vi "例7-4(2).vi"() -> ()   [LabVIEW 2019]
panel:
  in  "端口":dbl=65511.0
  out "波形图（客户机）":dbl[](graph)
  in  "停止按钮":bool
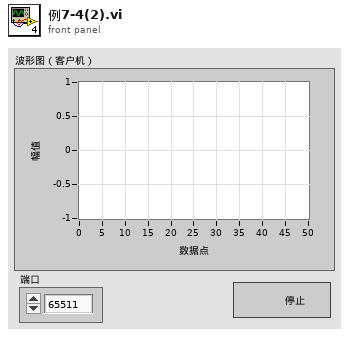
[diagram p1: front panel]
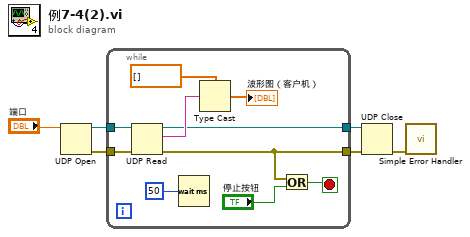
[diagram p0: block diagram]
diagram:
  n1 = UDP Open(11:"端口") -> (port=w6:refnum<k16>, 0:w5:errorcluster)  [unwired: 4 in, 1 out]
  n2 = while {
    tunnel: w6 -> [w16]
    tunnel: w5 -> [w15]
    tunnel: [w11] -> w3
    tunnel: [w8] -> w2
    stop <- w7 stop-if-true
    n3 = UDP Read(connection ID=w16, 8:w15) -> (data out=w14:string, error out=w8:errorcluster, 3:w11:refnum<k16>)  [unwired: 2 in, 2 out]
    n4 = Wait (ms)(milliseconds to wait=50) -> ()  [unwired: 1 out]
    n5 = Type Cast(type=dbl[] [], x=w14) -> (*(type *) &x=→"波形图（客户机）":dbl[])
    n6 = Or(x=w8, y="停止按钮") -> (x .or. y?=w7:bool)
  }
  n7 = UDP Close(connection ID=w3, 8:w2) -> (error out=w1:errorcluster)  [unwired: 1 out]
  n8 = call <vilib>:"Simple Error Handler.vi"("error in (no error)"=w1) -> ()  [unwired: 4 in, 5 out]
